vi "CreateWriter.vi"(4 "Is Colour":bool, 5 "Frames Per Second":dbl, 6 "Use HW":bool, 7 "Fourcc":T1, 8 "error in (no error)":errorcluster, 10 "Image Size":T2, 11 "Path":path) -> (0 "error out":errorcluster, 3 "Data Value Reference out":refnum<data-value>)   [LabVIEW 2020, in "video_io.lvlib"]
uses:
  video_io.lvlib
  common/Image Size (Integer).ctl
  FourCC.ctl
  common/common.lvlib
  common/bin/gartoolkit_videoio_32-1.dll
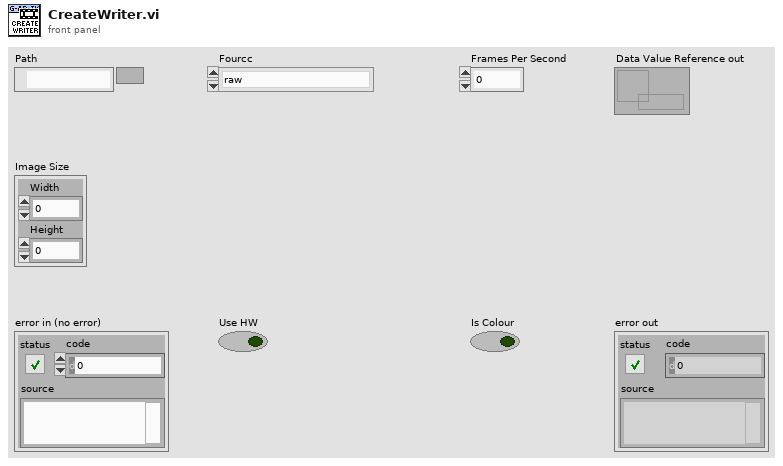
[diagram p1: front panel]
types:
  T1 = typedef "video_io.lvlib/FourCC.ctl" = enum16{"raw", "yuv2", "2vuy", "yuvs", "L555", "L565", "B565", "24BG", "BGRA", "RGBA", "ABGR", "b16g", "b48r", "bxbg", "bxrg", "bxyv", "NO16", "DVOO", "R420", "R411", "R10k", "R10g", "r210", "AVUI", "AVrp", "SUDS", "v210", "bxy2", "v308", "v408", "v410", "Y41P", "yuv4", "jpeg", "mjpa", "AVDJ", "AVRn", "dmb1", "mjpb", "SVQ1", "svq1", "svqi", "SVQ3", "mp4v", "DIVX", "XVID", "3IV2", "h263", "s263", "dvcp", "dvc", "dvpp", "dv5p", "dv5n", "AVdv", "AVd1", "dvhq", "dvhp", "dvh1", "dvh2", "dvh4", "dvh5", "dvh6", "dvh3", "VP31", "rpza", "cvid", "8BPS", "smc", "rle", "WRLE", "qdrw", "WRAW", "avc1", "ai5p", "ai5q", "ai52", "ai53", "ai55", "ai56", "ai1p", "ai1q", "ai12", "ai13", "ai15", "ai16", "m1v1", "mpeg", "m1v", "m2v1", "hdv1", "hdv2", "hdv3", "hdv4", "hdv5", "hdv6", "hdv7", "hdv8", "hdv9", "hdva", "mx5n", "mx5p", "mx4n", "mx4p", "mx3n", "mx3p", "xd54", "xd55", "xd59", "xd5a", "xd5b", "xd5c", "xd5d", "xd5e", "xd5f", "xdv1", "xdv2", "xdv3", "xdv4", "xdv5", "xdv6", "xdv7", "xdv8", "xdv9", "xdva", "xdvb", "xdvc", "xdvd", "xdve", "xdvf", "xdhd", "xdh2", "AVmp", "mjp2", "tga", "tiff", "gif", "png", "MNG", "vc-1", "avs2", "drac", "AVdn", "H263", "3IVD", "AV1x", "AVup", "sgi", "dpx", "exr", "apch", "apcn"}
  T2 = typedef "common.lvlib/Image Size (Integer).ctl" = cluster{"Width":u16, "Height":u16}
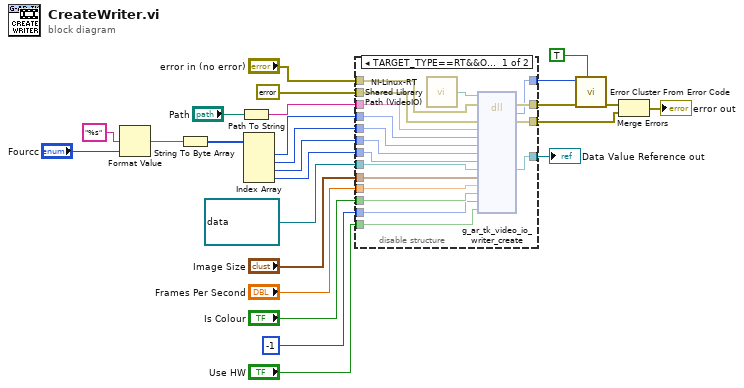
[diagram p0: block diagram]
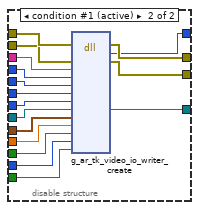
[diagram p2: hidden frame]
diagram:
  n1 = Format Value(format string="%s", value (0)="Fourcc") -> (output string=w2:string)  [unwired: 1 in]
  n2 = String To Byte Array(string=w2) -> (unsigned byte array=w16:u8[])
  n3 = Path To String(path="Path") -> (string=w14:string)
  n4 = Index Array(array=w16) -> (element #1=w17:u8, element #2=w18:u8, element #3=w19:u8, element #4=w20:u8)  [unwired: 4 in]
  n5 = disable-structure shown="TARGET_TYPE==RT&&OS==Linux" {
    disable-tunnel: "error in (no error)" -> [w43 w60]
    disable-tunnel: errorcluster {"status"=FALSE, "code"=0, "source"=""} ("error constant") -> [w41 w59]
    disable-tunnel: w14 -> [w40 w53]
    disable-tunnel: refnum<data-value> refnum ("EDVR") -> [w35 w58]
    disable-tunnel: [w29 w57] -> w9
    disable-tunnel: [w28 w56] -> w10
    disable-tunnel: [w30 w55] -> w25
    disable-tunnel: [w27 w54] -> w12
    disable-tunnel: w17 -> [w39 w52]
    disable-tunnel: w18 -> [w38 w51]
    disable-tunnel: w19 -> [w37 w50]
    disable-tunnel: w20 -> [w36 w49]
    disable-tunnel: "Image Size" -> [w34 w48]
    disable-tunnel: "Frames Per Second" -> [w33 w47]
    disable-tunnel: "Is Colour" -> [w32 w46]
    disable-tunnel: i8 -1 ("Quality") -> [w31 w45]
    disable-tunnel: "Use HW" -> [w26 w44]
    frame condition #0 {
      n6 = call "NI-Linux-RT Shared Library Path (VideoIO).vi"() -> ("Path"=w42:path)
      n7 = dll-call lib="?" fn="g_ar_tk_video_io_writer_create" ("g_ar_toolkit.*.*:g_ar_tk_capture_context_create")(path in=w42, error in=w43, "error_cluster"=w41, "Path"=w40, "fourcc_0"=w39, "fourrc_1"=w38, "fourcc_2"=w37, "fourcc_3"=w36, "Handle"=w35, "size"=w34, "fps"=w33, "is_colour"=w32, "quality"=w31, "use_harware_acc"=w26) -> (error out=w29:errorcluster, "return type"=w28:i32, "error_cluster"=w27:errorcluster, "Handle"=w30:refnum<data-value>)  [unwired: 11 in, 1 out]
    }
    frame condition #1 (active) {
      n8 = dll-call lib="C:/serenial/lib/g-augmented-reality-toolkit/LabVIEW/common/bin/gartoolkit_videoio_*-1.*" fn="g_ar_tk_video_io_writer_create" ("g_ar_toolkit.*.*:g_ar_tk_capture_context_create")(error in=w60, "error_cluster"=w59, "Path"=w53, "fourcc_0"=w52, "fourrc_1"=w51, "fourcc_2"=w50, "fourcc_3"=w49, "Handle"=w58, "size"=w48, "fps"=w47, "is_colour"=w46, "quality"=w45, "use_hw_acceleration"=w44) -> (error out=w57:errorcluster, "return type"=w56:i32, "error_cluster"=w54:errorcluster, "Handle"=w55:refnum<data-value>)  [unwired: 12 in, 1 out]
    }
  }
  "Data Value Reference out" <- w25
  n9 = call <vilib>:"Error Cluster From Error Code.vi"("show call chain? (False)"=TRUE, "error in (no error)"=w9, "error code (0)"=w10) -> ("error out"=w5:errorcluster)  [unwired: 6 in]
  n10 = Merge Errors(w5, w12) -> (→"error out":errorcluster)
